vi "enque.vi"(4 "timeout":dbl=1.0, 6 "data in":string, 8 "error in (no error)":errorcluster, 11 "py in":T1) -> (0 "error out":errorcluster, 1 "return value":string, 2 "response":T3, 3 "py out":T1)   [LabVIEW 2022 SP3, in "pythonq.lvlib"]
uses:
  pythonq.lvlib
  py_result.ctl
  py_session.ctl
  py_cluster.ctl
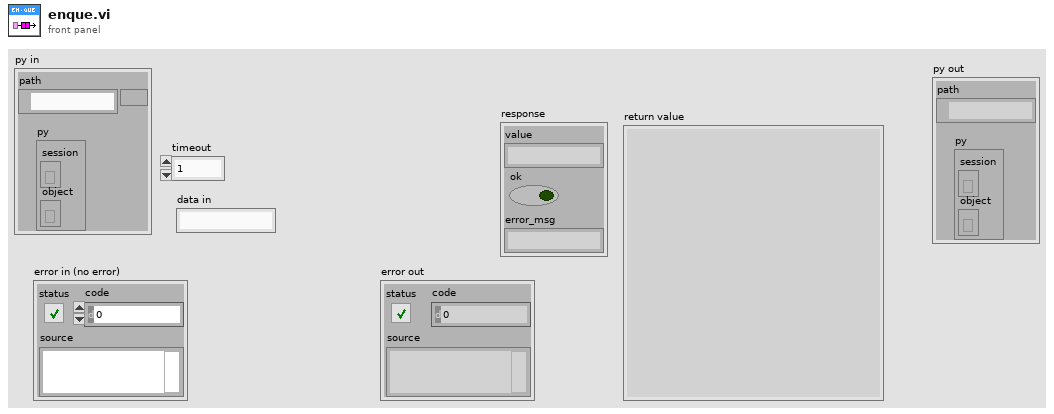
[diagram p1: front panel]
types:
  T1 = typedef "pythonq.lvlib/py_cluster.ctl" = cluster{"path":path, "py":T2}
  T2 = typedef "pythonq.lvlib/py_session.ctl" = cluster{"session":refnum<k35>, "object":refnum<k38>}
  T3 = typedef "pythonq.lvlib/py_result.ctl" = cluster{"value":string, "ok":bool, "error_msg":string}
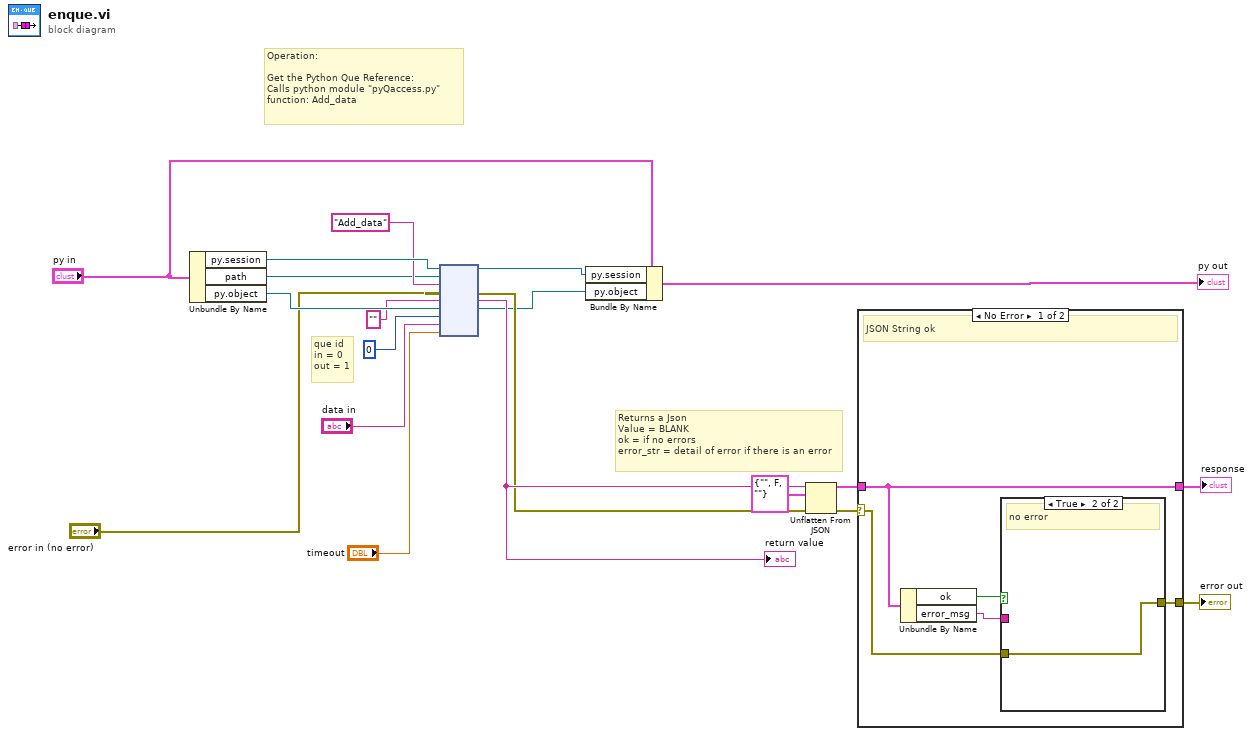
[diagram p0: block diagram]
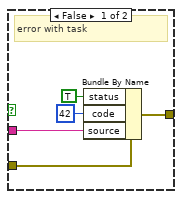
[diagram p2: hidden frame]
diagram:
  # "Returns a Json\nValue = BLANK\nok = if no errors\nerror_str = detail of error if there is an error"
  # "que id\nin = 0\nout = 1"
  # "Operation:\n\nGet the Python Que Reference:\nCalls python module \"pyQaccess.py\"\nfunction: Add_data"
  n1 = Unbundle By Name("py in") -> ("py.session"=w10:refnum<k35>, "path"=w5:path, "py.object"=w11:refnum<k38>)
  n2 = node(w10, w5, "Add_data" ("function name"), "error in (no error)", "", w11, 0, "data in", "timeout") -> (w7:refnum<k35>, w18:errorcluster, w20:string, w6:refnum<k38>)  [unwired: 3 in, 2 out]
  "return value" <- w20
  n3 = Bundle By Name(cluster="py in", "py.session"=w7, "py.object"=w6) -> (→"py out":T1)
  n4 = Unflatten From JSON(JSON string=w20, type and defaults=T3 {"value"="", "ok"=FALSE, "error_msg"=""}, error in (no error)=w18) -> (value=w17:T3, error out=w16:errorcluster)  [unwired: 4 in]
  n5 = case shown="No Error" w16 {
    selector: w16 -> [w23 w32]
    tunnel: w17 -> [w25 w33]
    tunnel: [w25 w33] -> w15
    tunnel: [w22 w32] -> w14
    frame No Error {
      # "JSON String ok"
      n6 = Unbundle By Name(w25) -> ("ok"=w24:bool, "error_msg"=w21:string)
      n7 = case shown="True" w24 {
        tunnel: w23 -> [w30 w31]
        tunnel: [w28 w31] -> w22
        tunnel: w21 -> [w27 _]
        frame False {
          # "error with task"
          n8 = Bundle By Name(cluster=w30, "status"=TRUE, "code"=42, "source"=w27) -> (w28:errorcluster)
        }
        frame True {
          # "no error"
        }
      }
    }
    frame Error {
    }
  }
  "error out" <- w14
  "response" <- w15
